vi "NIIE_Rectangle.vi"(6 "Fill Color":u32(colorbox), 7 "Fill?(F)":bool, 8 "Error":errorcluster, 9 "Edge Color":u32(colorbox), 11 "Rect":T1) -> (0 "Error Out":errorcluster, 3 "New Picture Out":picture)   [LabVIEW 2021]
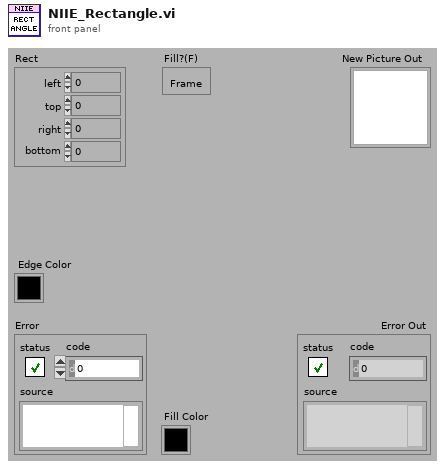
[diagram p1: front panel]
types:
  T1 = cluster{"left":i16, "top":i16, "right":i16, "bottom":i16}
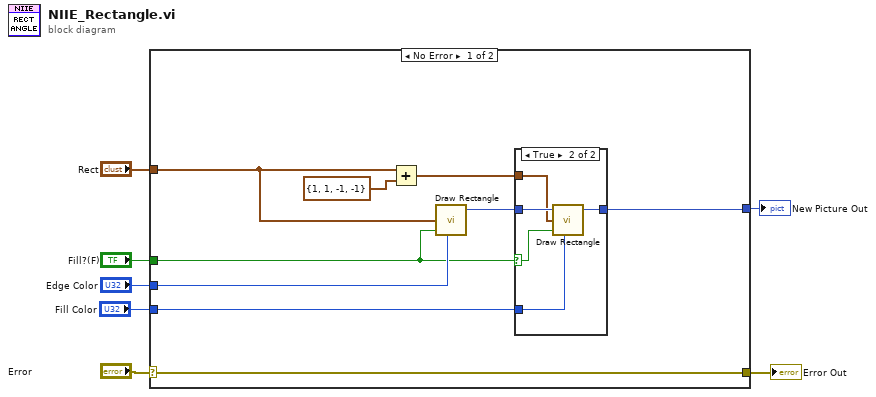
[diagram p0: block diagram]
diagram:
  n1 = case shown="No Error" "Error" {
    selector: "Error" -> [w16 w23]
    tunnel: [w16 w23] -> w6
    tunnel: [w10 _] -> w5
    tunnel: "Rect" -> [w13 _]
    tunnel: "Edge Color" -> [w15 _]
    tunnel: "Fill?(F)" -> [w12 _]
    tunnel: "Fill Color" -> [w8 _]
    frame No Error {
      n2 = Add(x=w13, y=T1 {"left"=1, "top"=1, "right"=-1, "bottom"=-1}) -> (x+y=w9:T1)
      n3 = call <vilib>:"Draw Rectangle.vi"("rect"=w13, "fill?(F)"=w12, "color(black)"=w15) -> ("new picture"=w11:picture)  [unwired: 6 in]
      n4 = case shown="True" w12 {
        selector: w12 -> [_ w19]
        tunnel: w11 -> [w17 w22]
        tunnel: [w17 w21] -> w10
        tunnel: w9 -> [_ w20]
        tunnel: w8 -> [_ w18]
        frame False {
        }
        frame True {
          n5 = call <vilib>:"Draw Rectangle.vi"("picture"=w22, "rect"=w20, "fill?(F)"=w19, "color(black)"=w18) -> ("new picture"=w21:picture)  [unwired: 5 in]
        }
      }
    }
    frame Error {
    }
  }
  "Error Out" <- w6
  "New Picture Out" <- w5
